vi "Planner_Creator.vi"(8 "error in (no error)":errorcluster) -> (0 "error out":errorcluster)   [LabVIEW 2017]
uses:
  <vilib>/Utility/file.llb/Read Delimited Spreadsheet (string).vi
  <vilib>/Utility/file.llb/Write Delimited Spreadsheet (string).vi
  <vilib>/Utility/config.llb/NI_LVConfig.lvlib
panel:
  out "SECTION 2":T1
  out "SECTION 1":T2
  in  "SECTION No":string(combo)
  in  "Delete Button":bool
  in  "Save Button":bool
  in  "Qty":u16=1 min=1 max=90 step=1
  in  "HOME":bool
  in  "UPDATE TABLE":bool
  in  "FG CAT No":string(combo)
  # "Plan Creater"
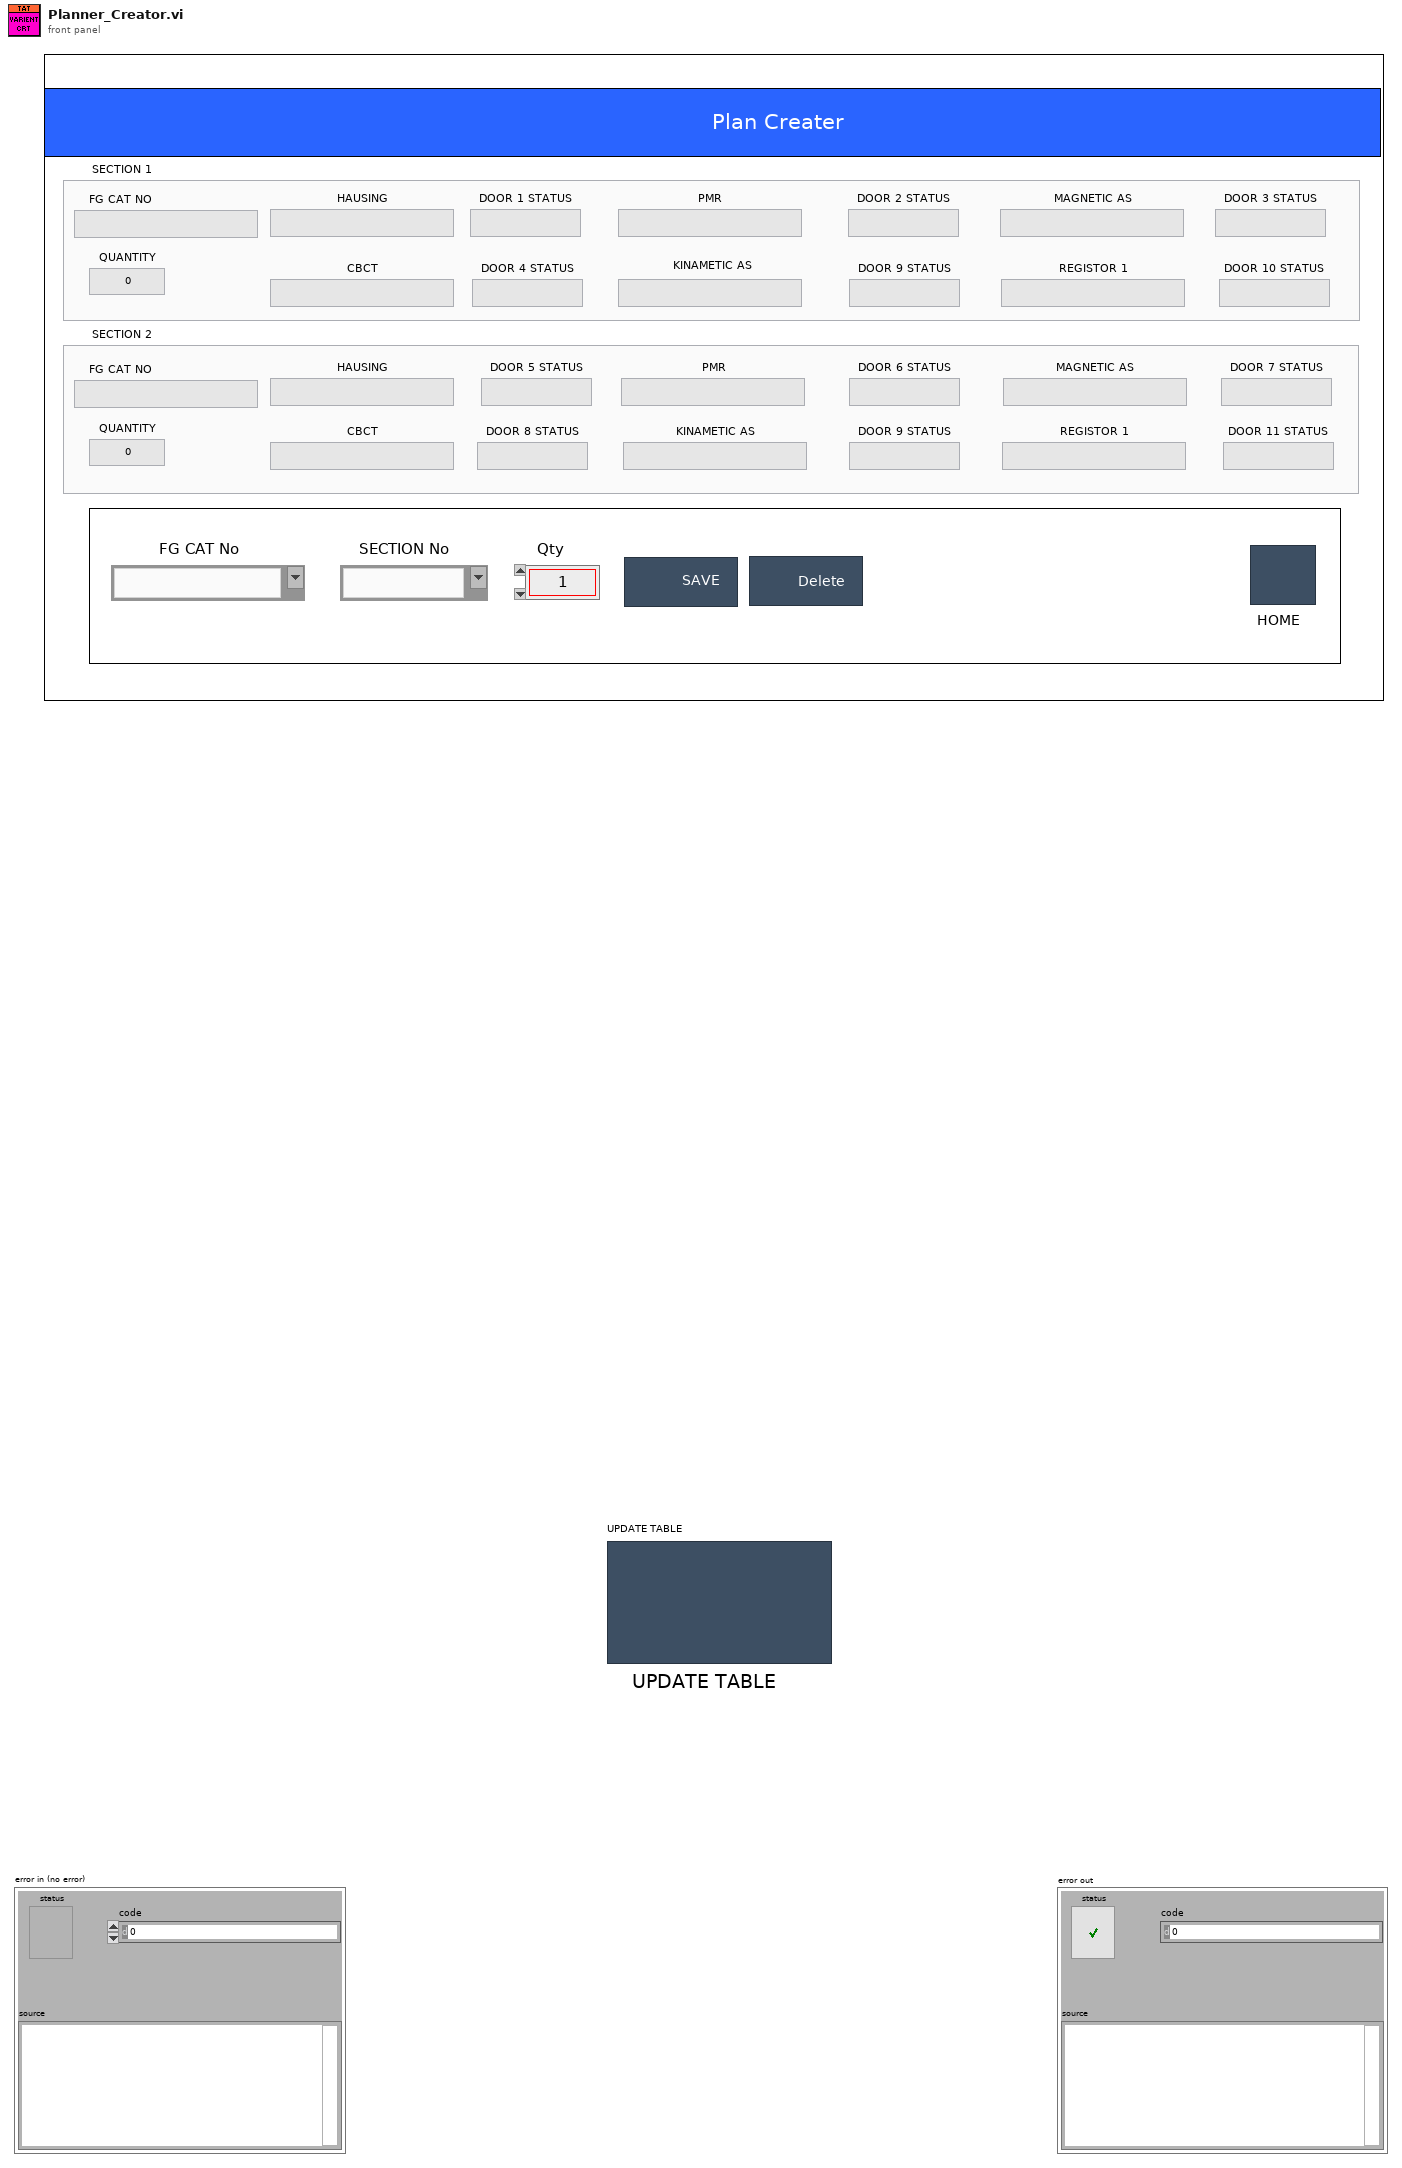
[diagram p1: front panel]
types:
  T1 = cluster{"FG CAT NO":string, "HAUSING":string, "DOOR 5 STATUS":string, "PMR":string, "DOOR 6 STATUS":string, "MAGNETIC AS":string, "DOOR 7 STATUS":string, "CBCT":string, "DOOR 8 STATUS":string, "KINAMETIC AS":string, "DOOR 9 STATUS":string, "REGISTOR 1":string, "DOOR 11 STATUS":string, "QUANTITY":u16}
  T2 = cluster{"FG CAT NO":string, "HAUSING":string, "DOOR 1 STATUS":string, "PMR":string, "DOOR 2 STATUS":string, "MAGNETIC AS":string, "DOOR 3 STATUS":string, "CBCT":string, "DOOR 4 STATUS":string, "KINAMETIC AS":string, "DOOR 9 STATUS":string, "REGISTOR 1":string, "DOOR 10 STATUS":string, "QUANTITY":u16}
  T3 = enum32{"invalid app kind", "Development System", "Run Time System", "Student Edition", "Embedded LabVIEW", "Evaluation", "Custom"}
  T4 = typedef "NI_LVConfig.lvlib/Config Data RefNum.ctl" = refnum<k1>
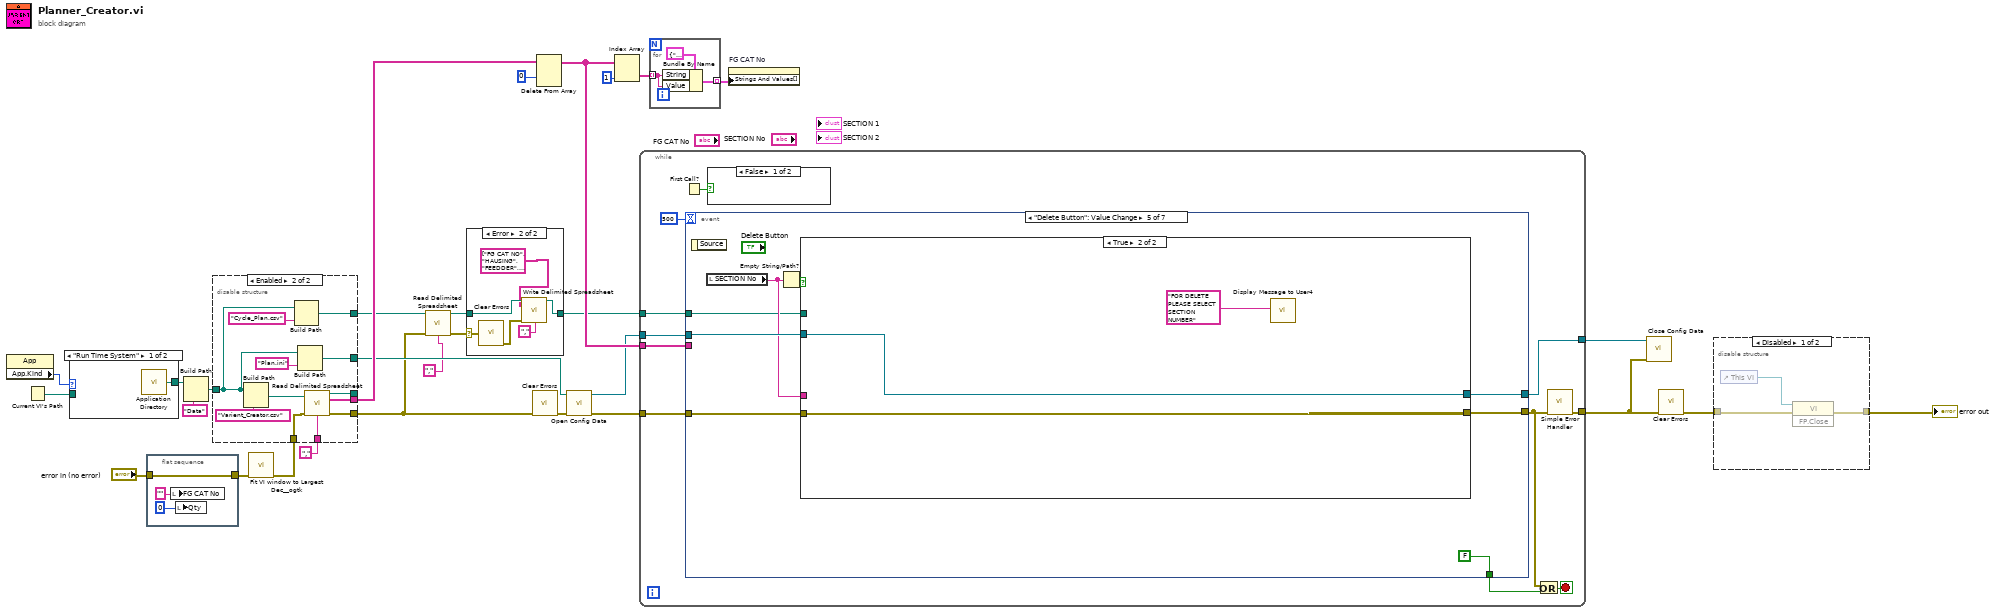
[diagram p0: block diagram]
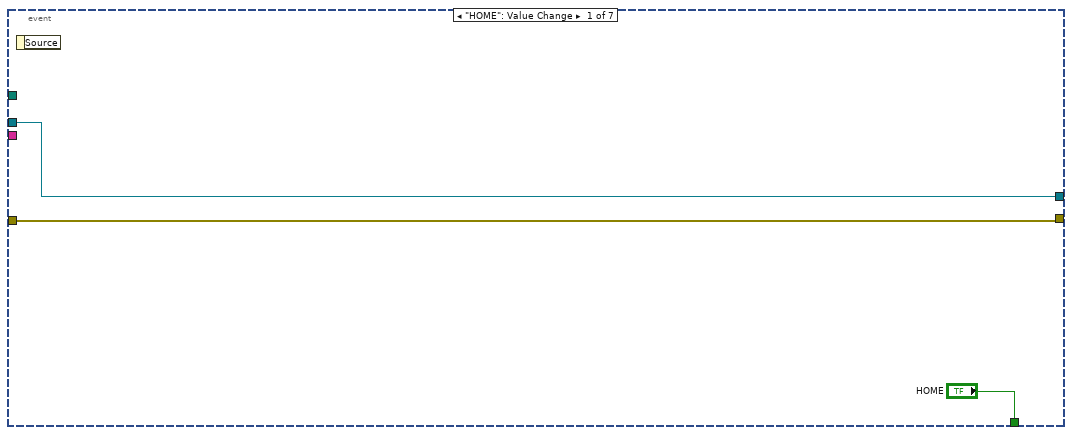
[diagram p4: hidden frame]
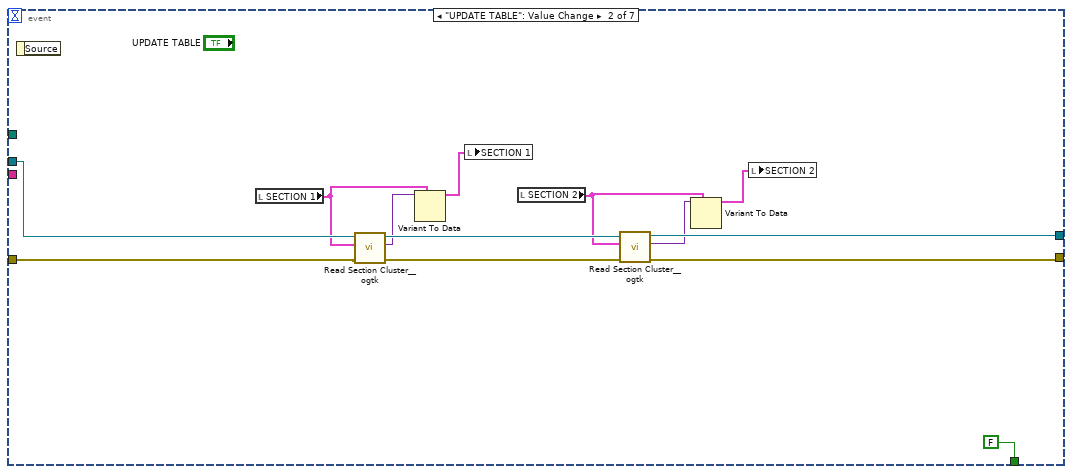
[diagram p5: hidden frame]
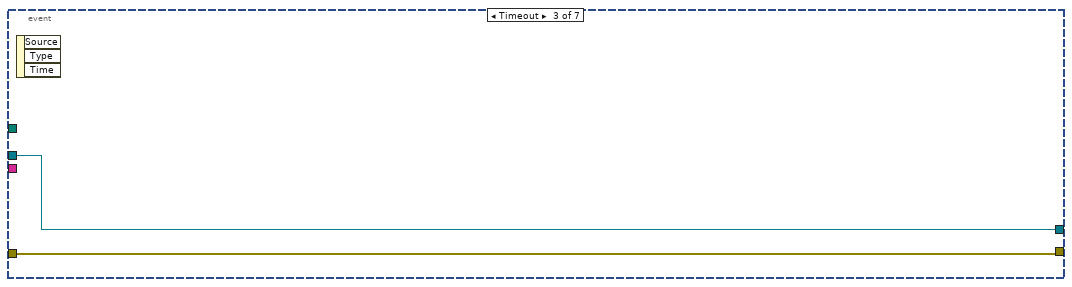
[diagram p6: hidden frame]
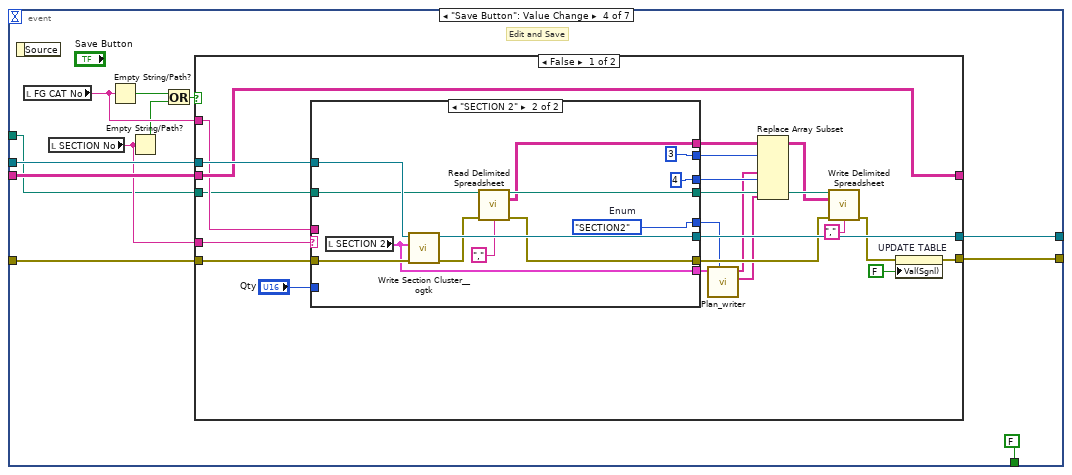
[diagram p7: hidden frame]
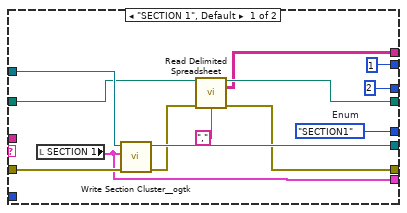
[diagram p8: hidden frame]
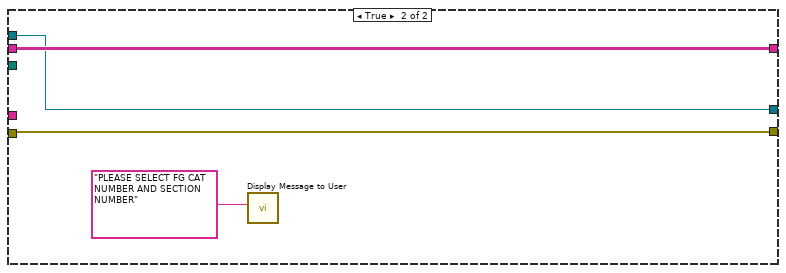
[diagram p9: hidden frame]
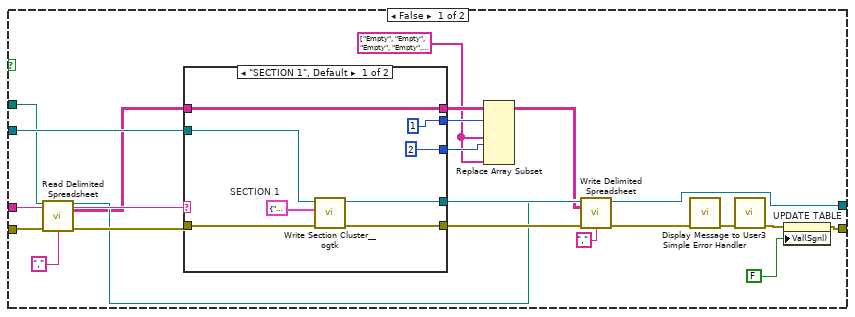
[diagram p10: hidden frame]
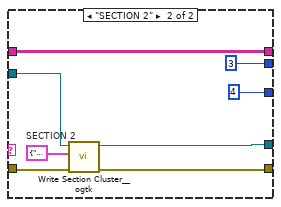
[diagram p11: hidden frame]
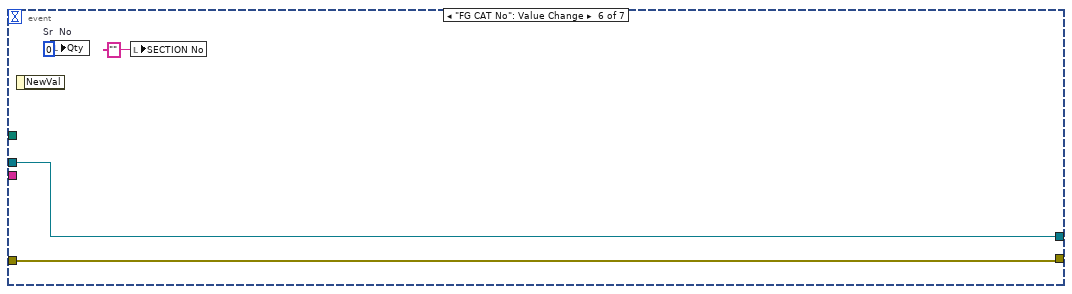
[diagram p12: hidden frame]
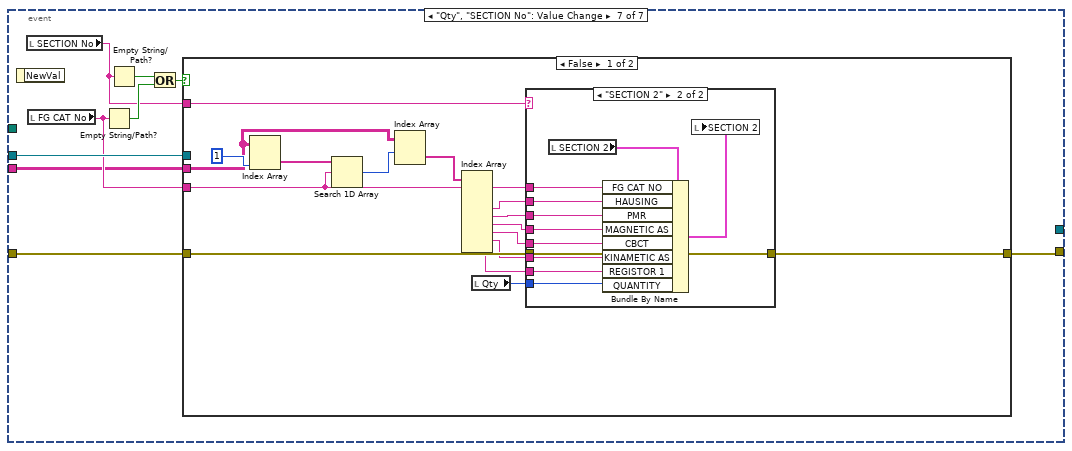
[diagram p13: hidden frame]
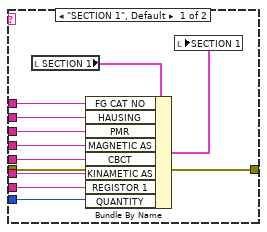
[diagram p14: hidden frame]
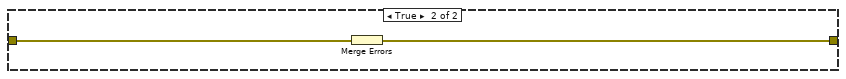
[diagram p15: hidden frame]
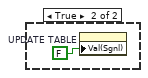
[diagram p16: hidden frame]
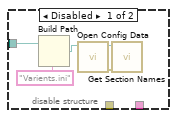
[diagram p17: hidden frame]
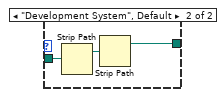
[diagram p18: hidden frame]
diagram:
  n1 = property class="App"() -> ("App.Kind"=w23:T3)  [unwired: 2 in, 2 out]
  n2 = Current VI's Path() -> (path=w24:path)
  n3 = case shown="\"Run Time System\"" w23 {
    tunnel: w24 -> [_ w32]
    tunnel: [w30 w31] -> w20
    frame "Run Time System" {
      n4 = call <vilib>:"Application Directory.vi"() -> ("Application Directory"=w30:path)
    }
    frame "Development System", Default {
      n5 = Strip Path(path=w32) -> (stripped path=w33:path)  [unwired: 1 out]
      n6 = Strip Path(path=w33) -> (stripped path=w31:path)  [unwired: 1 out]
    }
  }
  n7 = flat-sequence {
    tunnel: [w36] -> w25
    tunnel: "error in (no error)" -> [w36]
    frame #0 {
      n8 = local write "FG CAT No"("" ("PART NUMBER")) -> ()
      n9 = local write "Qty"(u16 0 ("BATCH SIZE")) -> ()
    }
  }
  n10 = Build Path(base path=w20, name or relative path="Data") -> (appended path=w21:path)
  n11 = call <userlib>:"Fit VI window to Largest Dec__ogtk.vi"("error in (no error)"=w25) -> ("error out"=w19:errorcluster)  [unwired: 5 in, 1 out]
  n12 = disable-structure shown="Enabled" {
    disable-tunnel: w21 -> [w37 w43]
    disable-tunnel: w19 -> [_ w51]
    disable-tunnel: [_ w50] -> w17
    disable-tunnel: [_ w49] -> _
    disable-tunnel: [_ w48] -> w6
    disable-tunnel: "," -> [_ w47]
    disable-tunnel: [_ w45] -> w11
    disable-tunnel: [_ w42] -> w5
    frame Disabled {
      n13 = Build Path(base path=w37, name or relative path="Varients.ini") -> (appended path=w41:path)
      n14 = call <vilib>:"Open Config Data.vi"("configuration file path"=w41) -> ("error out"=w38:errorcluster, "refnum"=w39:T4)  [unwired: 8 in, 1 out]
      n15 = call <vilib>:"Get Section Names.vi"("error in (no error)"=w38, "refnum"=w39) -> ()  [unwired: 7 in, 3 out]
    }
    frame Enabled {
      n16 = Build Path(base path=w43, name or relative path="Varient_Creator.csv") -> (appended path=w52:path)
      n17 = Build Path(base path=w43, name or relative path="Cycle_Plan.csv") -> (appended path=w42:path)
      n18 = Build Path(base path=w43, name or relative path="Plan.ini") -> (appended path=w45:path)
      n19 = call-poly <vilib>:"Read Delimited Spreadsheet.vi"("file path (dialog if empty)"=w52, "error in (no error)"=w51, "delimiter (\\t)"=w47) -> ("new file path (Not A Path if cancelled)"=w49:path, "all rows"=w50:string[][], "error out"=w48:errorcluster)  [unwired: 7 in, 3 out]
    }
  }
  n20 = call-poly <vilib>:"Read Delimited Spreadsheet.vi"("file path (dialog if empty)"=w5, "error in (no error)"=w6, "delimiter (\\t)"=",") -> ("new file path (Not A Path if cancelled)"=w1:path, "error out"=w3:errorcluster)  [unwired: 7 in, 4 out]
  n21 = case shown="Error" w3 {
    selector: w3 -> [_ w57]
    tunnel: [w54 w58] -> w2
    tunnel: w1 -> [w54 w59]
    frame No Error {
    }
    frame Error {
      n22 = call <vilib>:"Clear Errors.vi"("error in (no error)"=w57) -> ("error out"=w56:errorcluster)  [unwired: 5 in, 1 out]
      n23 = call-poly <vilib>:"Write Delimited Spreadsheet.vi"("file path (dialog if empty)"=w59, "2D data"=string[][] [["FG CAT NO", "HAUSING", "FEEDDER", "HAUSING_QR_CODE", "DOOR", "PMR", "FEEDDER", "PMR_QR_CODE", "DOOR", "MAGNETIC AS", "FEEDDER", "MAGNETIC AS_QR_CODE", "DOOR", "CBCT", "FEEDDER", "CBCT_QR_CODE", "DOOR", "KINAMETIC AS", "FEEDDER", "KINAMETIC AS_QR_CODE", "DOOR", "REGISTOR 1", "FEEDDER", "REGISTOR 1_QR_CODE", "DOOR", "QTY", "QTY_DONE"], ["Empty", "Empty", "Empty", "Empty", "Empty", "Empty", "Empty", "Empty", "Empty", "Empty", "Empty", "Empty", "Empty", "Empty", "Empty", "Empty", "Empty", "Empty", "Empty", "Empty", "Empty", "Empty", "Empty", "Empty", "Empty", "Empty", "Empty"], ["Empty", "Empty", "Empty", "Empty", "Empty", "Empty", "Empty", "Empty", "Empty", "Empty", "Empty", "Empty", "Empty", "Empty", "Empty", "Empty", "Empty", "Empty", "Empty", "Empty", "Empty", "Empty", "Empty", "Empty", "Empty", "Empty", "Empty"], ["Empty", "Empty", "Empty", "Empty", "Empty", "Empty", "Empty", "Empty", "Empty", "Empty", "Empty", "Empty", "Empty", "Empty", "Empty", "Empty", "Empty", "Empty", "Empty", "Empty", "Empty", "Empty", "Empty", "Empty", "Empty", "Empty", "Empty"], ["Empty", "Empty", "Empty", "Empty", "Empty", "Empty", "Empty", "Empty", "Empty", "Empty", "Empty", "Empty", "Empty", "Empty", "Empty", "Empty", "Empty", "Empty", "Empty", "Empty", "Empty", "Empty", "Empty", "Empty", "Empty", "Empty", "Empty"]], "error in (no error)"=w56, "delimiter (\\t)"=",") -> ("new file path (Not A Path if cancelled)"=w58:path)  [unwired: 10 in, 1 out]
    }
  }
  n24 = call <vilib>:"Clear Errors.vi"("error in (no error)"=w6) -> ("error out"=w9:errorcluster)  [unwired: 5 in, 1 out]
  n25 = Delete From Array(array=w17, index (row)=0) -> (array with subset deleted=w12:string[][])  [unwired: 2 in, 1 out]
  n26 = call <vilib>:"Open Config Data.vi"("error in (no error)"=w9, "configuration file path"=w11) -> ("error out"=w8:errorcluster, "refnum"=w10:T4)  [unwired: 7 in, 1 out]
  n27 = Index Array(array=w12, index (col)=1) -> (element=w14:string[])  [unwired: 1 in]
  n28 = while {
    tunnel: [w66] -> w27
    tunnel: w8 -> [w68]
    tunnel: w12 -> [w64]
    tunnel: w10 -> [w63]
    tunnel: [w62] -> w7
    tunnel: w2 -> [w61]
    stop <- w70 stop-if-true
    n29 = First Call?() -> (First Call?: T/F=w69:bool)
    n30 = event shown="[4] \"Delete Button\": Value Change" {
      selector: _ -> [_ _ _ _ _ _ _]
      dyn-events: _ -> [_ _ _ _ _ _ _]
      timeout: 500 -> [_ _ _ _ _ _ _]
      tunnel: ["HOME" FALSE ("stop") _ FALSE ("stop") FALSE ("stop") _ _] -> w71
      tunnel: [w73 w84 w89 w99 w159 w204 w213] -> w67
      tunnel: w68 -> [w73 w85 w89 w98 w158 w204 w214]
      tunnel: w64 -> [_ _ _ w97 _ _ w206]
      tunnel: w63 -> [w72 w82 w88 w93 w157 w202 w209]
      tunnel: [w72 w81 w88 w91 w156 w202 _] -> w62
      tunnel: w61 -> [_ _ _ w90 w154 _ _]
      event "HOME": Value Change {
        n31 = event-data() -> ()  [unwired: 1 in, 1 out]
      }
      event "UPDATE TABLE": Value Change {
        n32 = event-data() -> ()  [unwired: 1 in, 1 out]
        n33 = local read "SECTION 1"() -> (w80:T2)
        n34 = call <userlib>:"Read Section Cluster__ogtk.vi"("error in (no error)"=w85, "Section Formatted Cluster Type"=w80, "refnum"=w82) -> ("error out"=w86:errorcluster, "Section Formatted Cluster"=w79:variant, "dup refnum"=w83:T4)  [unwired: 4 in, 2 out]
        n35 = Variant To Data(type=w80, Variant=w79) -> (data=w75:T2)  [unwired: 1 in, 1 out]
        n36 = local write "SECTION 1"(w75) -> ()
        n37 = local read "SECTION 2"() -> (w78:T1)
        n38 = call <userlib>:"Read Section Cluster__ogtk.vi"("error in (no error)"=w86, "Section Formatted Cluster Type"=w78, "refnum"=w83) -> ("error out"=w84:errorcluster, "Section Formatted Cluster"=w77:variant, "dup refnum"=w81:T4)  [unwired: 4 in, 2 out]
        n39 = Variant To Data(type=w78, Variant=w77) -> (data=w76:T1)  [unwired: 1 in, 1 out]
        n40 = local write "SECTION 2"(w76) -> ()
      }
      event Timeout {
        n41 = event-data() -> ()  [unwired: 1 in, 3 out]
      }
      event "Save Button": Value Change {
        # "Edit and Save"
        n42 = event-data() -> ()  [unwired: 1 in, 1 out]
        n43 = local read "FG CAT No"() -> (w100:string)
        n44 = local read "SECTION No"() -> (w92:string)
        n45 = Empty String/Path?(string/path=w100) -> (empty?=w95:bool)
        n46 = Empty String/Path?(string/path=w92) -> (empty?=w96:bool)
        n47 = Or(x=w95, y=w96) -> (x .or. y?=w94:bool)
        n48 = case shown="False" w94 {
          tunnel: [w122 w152] -> w99
          tunnel: w100 -> [w118 _]
          tunnel: w98 -> [w120 w152]
          tunnel: w97 -> [w119 w151]
          tunnel: w93 -> [w121 w150]
          tunnel: [w119 w151] -> _
          tunnel: w92 -> [w117 _]
          tunnel: [w115 w150] -> w91
          tunnel: w90 -> [w114 _]
          frame False {
            n49 = case shown="\"SECTION 2\"" w117 {
              tunnel: w121 -> [w135 w148]
              tunnel: w120 -> [w136 w147]
              tunnel: [w130 w145] -> w112
              tunnel: w118 -> [_ _]
              tunnel: "Qty" -> [_ _]
              tunnel: [w134 w149] -> w115
              tunnel: w114 -> [w132 w144]
              tunnel: [w129 w143] -> w113
              tunnel: [w128 w141] -> w109
              tunnel: [1 ("disabled index (col)") 3 ("disabled index (col)")] -> w107
              tunnel: [2 ("disabled index (col)") 4 ("disabled index (col)")] -> w106
              tunnel: [w125 w138] -> w105
              tunnel: [w124 w137] -> w102
              frame "SECTION 1", Default {
                w124 = enum16{"SECTION1", "SECTION2"}."SECTION1"  # Enum
                n50 = local read "SECTION 1"() -> (w125:T2)
                n51 = call <userlib>:"Write Section Cluster__ogtk.vi"("error in (no error)"=w136, "Section Formatted Cluster"=w125, "refnum"=w135) -> ("error out"=w131:errorcluster, "dup refnum"=w134:T4)  [unwired: 7 in]
                n52 = call-poly <vilib>:"Read Delimited Spreadsheet.vi"("file path (dialog if empty)"=w132, "error in (no error)"=w131, "delimiter (\\t)"=",") -> ("new file path (Not A Path if cancelled)"=w129:path, "all rows"=w128:string[][], "error out"=w130:errorcluster)  [unwired: 7 in, 3 out]
              }
              frame "SECTION 2" {
                w137 = enum16{"SECTION1", "SECTION2"}."SECTION2"  # Enum
                n53 = local read "SECTION 2"() -> (w138:T1)
                n54 = call <userlib>:"Write Section Cluster__ogtk.vi"("error in (no error)"=w147, "Section Formatted Cluster"=w138, "refnum"=w148) -> ("error out"=w146:errorcluster, "dup refnum"=w149:T4)  [unwired: 7 in]
                n55 = call-poly <vilib>:"Read Delimited Spreadsheet.vi"("file path (dialog if empty)"=w144, "error in (no error)"=w146, "delimiter (\\t)"=",") -> ("new file path (Not A Path if cancelled)"=w143:path, "all rows"=w141:string[][], "error out"=w145:errorcluster)  [unwired: 7 in, 3 out]
              }
            }
            n56 = call "Plan_writer.vi"("Enum"=w102, "SECTION IN"=w105) -> ("Section Second 45"=w103:string[], "Section first 45"=w104:string[])  [unwired: 8 in]
            n57 = Replace Array Subset(array=w109, new element #1=w104, index (row) #1=w107, new element #2=w103, index (row) #2=w106) -> (w108:string[][])  [unwired: 2 in]
            n58 = call-poly <vilib>:"Write Delimited Spreadsheet.vi"("file path (dialog if empty)"=w113, "2D data"=w108, "error in (no error)"=w112, "delimiter (\\t)"=",") -> ("error out"=w111:errorcluster)  [unwired: 10 in, 1 out]
            n59 = property on="UPDATE TABLE" class="Bool (strict)"(error in=w111, "Val(Sgnl)"=FALSE) -> (error out=w122:errorcluster)  [unwired: 1 in, 1 out]
          }
          frame True {
            n60 = call "Display Message to User"("Message"="PLEASE SELECT FG CAT NUMBER AND SECTION NUMBER") -> ()  [unwired: 9 in, 2 out]
          }
        }
      }
      event "Delete Button": Value Change {
        n61 = event-data() -> ()  [unwired: 1 in, 1 out]
        n62 = local read "SECTION No"() -> (w155:string)
        n63 = Empty String/Path?(string/path=w155) -> (empty?=w160:bool)
        n64 = case shown="True" w160 {
          tunnel: [w181 w200] -> w159
          tunnel: w158 -> [w175 w200]
          tunnel: w157 -> [w178 w199]
          tunnel: [w177 w199] -> w156
          tunnel: w155 -> [w176 _]
          tunnel: w154 -> [w172 _]
          frame False {
            w163 = string[] ["Empty", "Empty", "Empty", "Empty", "Empty", "Empty", "Empty", "Empty", "Empty", "Empty", "Empty", "Empty", "Empty", "Empty", "Empty", "Empty", "Empty", "Empty", "Empty", "Empty", "Empty", "Empty", "Empty", "Empty", "Empty", "Empty", "Empty"]
            n65 = call-poly <vilib>:"Read Delimited Spreadsheet.vi"("file path (dialog if empty)"=w172, "error in (no error)"=w175, "delimiter (\\t)"=",") -> ("new file path (Not A Path if cancelled)"=w168:path, "all rows"=w166:string[][], "error out"=w174:errorcluster)  [unwired: 7 in, 3 out]
            n66 = case shown="\"SECTION 1\", Default" w176 {
              tunnel: w174 -> [w190 w196]
              tunnel: [w189 w198] -> w170
              tunnel: [w188 w197] -> w177
              tunnel: w178 -> [w187 w195]
              tunnel: [w185 w193] -> w167
              tunnel: w166 -> [w185 w193]
              tunnel: [1 ("disabled index (col)") 3 ("disabled index (col)")] -> w165
              tunnel: [2 ("disabled index (col)") 4 ("disabled index (col)")] -> w164
              frame "SECTION 1", Default {
                w186 = T2 {"FG CAT NO"="", "HAUSING"="", "DOOR 1 STATUS"="PENDING", "PMR"="", "DOOR 2 STATUS"="PENDING", "MAGNETIC AS"="", "DOOR 3 STATUS"="PENDING", "CBCT"="", "DOOR 4 STATUS"="PENDING", "KINAMETIC AS"="", "DOOR 9 STATUS"="PENDING", "REGISTOR 1"="", "DOOR 10 STATUS"="PENDING", "QUANTITY"=0}  # SECTION 1
                n67 = call <userlib>:"Write Section Cluster__ogtk.vi"("error in (no error)"=w190, "Section Formatted Cluster"=w186, "refnum"=w187) -> ("error out"=w189:errorcluster, "dup refnum"=w188:T4)  [unwired: 7 in]
              }
              frame "SECTION 2" {
                w194 = T1 {"FG CAT NO"="", "HAUSING"="", "DOOR 5 STATUS"="PENDING", "PMR"="", "DOOR 6 STATUS"="PENDING", "MAGNETIC AS"="", "DOOR 7 STATUS"="PENDING", "CBCT"="", "DOOR 8 STATUS"="PENDING", "KINAMETIC AS"="", "DOOR 9 STATUS"="PENDING", "REGISTOR 1"="", "DOOR 11 STATUS"="PENDING", "QUANTITY"=0}  # SECTION 2
                n68 = call <userlib>:"Write Section Cluster__ogtk.vi"("error in (no error)"=w196, "Section Formatted Cluster"=w194, "refnum"=w195) -> ("error out"=w198:errorcluster, "dup refnum"=w197:T4)  [unwired: 7 in]
              }
            }
            n69 = Replace Array Subset(array=w167, new element #1=w163, index (row) #1=w165, new element #2=w163, index (row) #2=w164) -> (w162:string[][])  [unwired: 2 in]
            n70 = call-poly <vilib>:"Write Delimited Spreadsheet.vi"("file path (dialog if empty)"=w168, "2D data"=w162, "error in (no error)"=w170, "delimiter (\\t)"=",") -> ("error out"=w169:errorcluster)  [unwired: 10 in, 1 out]
            n71 = call <vilib>:"Simple Error Handler.vi"("error in (no error)"=w169) -> ("error out"=w180:errorcluster)  [unwired: 4 in, 4 out]
            n72 = call "Display Message to User3"("error in (no error)"=w180) -> ("error out"=w179:errorcluster)  [unwired: 9 in, 1 out]
            n73 = property on="UPDATE TABLE" class="Bool (strict)"(error in=w179, "Val(Sgnl)"=FALSE) -> (error out=w181:errorcluster)  [unwired: 1 in, 1 out]
          }
          frame True {
            n74 = call "Display Message to User4"("Message"="FOR DELETE PLEASE SELECT SECTION NUMBER") -> ()  [unwired: 9 in, 2 out]
          }
        }
      }
      event "FG CAT No": Value Change {
        w205 = u16 0  # Sr  No
        n75 = event-data() -> ()  [unwired: 1 in, 1 out]
        n76 = local write "Qty"(w205) -> ()
        n77 = local write "SECTION No"("") -> ()
      }
      event "Qty", "SECTION No": Value Change {
        n78 = event-data() -> ()  [unwired: 1 in, 1 out]
        n79 = local read "SECTION No"() -> (w207:string)
        n80 = local read "FG CAT No"() -> (w208:string)
        n81 = Empty String/Path?(string/path=w208) -> (empty?=w211:bool)
        n82 = Empty String/Path?(string/path=w207) -> (empty?=w212:bool)
        n83 = Or(x=w212, y=w211) -> (x .or. y?=w210:bool)
        n84 = case shown="False" w210 {
          tunnel: w214 -> [w230 w254]
          tunnel: [w229 w253] -> w213
          tunnel: w209 -> [_ _]
          tunnel: w207 -> [w228 _]
          tunnel: w208 -> [w225 _]
          tunnel: w206 -> [w222 _]
          frame False {
            n85 = Index Array(array=w222, index (col)=1) -> (element=w224:string[])  [unwired: 1 in]
            n86 = Search 1D Array(1D array=w224, element=w225) -> (index of element=w223:i32)  [unwired: 1 in]
            n87 = Index Array(array=w222, index (row)=w223) -> (element=w221:string[])  [unwired: 1 in]
            n88 = Index Array(array=w221) -> (element #3=w220:string, element #4=w219:string, element #5=w218:string, element #6=w217:string, element #7=w216:string, element #8=w215:string)  [unwired: 8 in, 2 out]
            n89 = local read "Qty"() -> (w227:u16)
            n90 = case shown="\"SECTION 2\"" w228 {
              tunnel: w230 -> [w241 w252]
              tunnel: [w241 w252] -> w229
              tunnel: w225 -> [w239 w248]
              tunnel: w227 -> [w238 w249]
              tunnel: w220 -> [w231 w247]
              tunnel: w219 -> [w232 w246]
              tunnel: w218 -> [w233 w245]
              tunnel: w217 -> [w234 w244]
              tunnel: w216 -> [w235 w243]
              tunnel: w215 -> [w236 w242]
              frame "SECTION 1", Default {
                n91 = local read "SECTION 1"() -> (w240:T2)
                n92 = Bundle By Name(cluster=w240, "FG CAT NO"=w239, "HAUSING"=w231, "PMR"=w232, "MAGNETIC AS"=w233, "CBCT"=w234, "KINAMETIC AS"=w235, "REGISTOR 1"=w236, "QUANTITY"=w238) -> (w237:T2)
                n93 = local write "SECTION 1"(w237) -> ()
              }
              frame "SECTION 2" {
                n94 = local read "SECTION 2"() -> (w251:T1)
                n95 = Bundle By Name(cluster=w251, "FG CAT NO"=w248, "HAUSING"=w247, "PMR"=w246, "MAGNETIC AS"=w245, "CBCT"=w244, "KINAMETIC AS"=w243, "REGISTOR 1"=w242, "QUANTITY"=w249) -> (w250:T1)
                n96 = local write "SECTION 2"(w250) -> ()
              }
            }
          }
          frame True {
            n97 = Merge Errors(w254) -> (w253:errorcluster)
          }
        }
      }
    }
    n98 = case shown="False" w69 {
      frame False {
      }
      frame True {
        n99 = property on="UPDATE TABLE" class="Bool (strict)"("Val(Sgnl)"=FALSE) -> ()  [unwired: 2 in, 2 out]
      }
    }
    n100 = Or(x=w67, y=w71) -> (x .or. y?=w70:bool)
    n101 = call <vilib>:"Simple Error Handler.vi"("error in (no error)"=w67) -> ("error out"=w66:errorcluster)  [unwired: 4 in, 4 out]
  }
  n102 = for {
    tunnel: w14 -> [w257] mode=indexing
    tunnel: [w256] -> w13 mode=indexing
    n103 = Bundle By Name(cluster=cluster{"String":string, "Value":string} {"String"="", "Value"=""}, "String"=w257, "Value"=w257) -> (w256:cluster{"String":string, "Value":string})
  }
  n104 = property on="FG CAT No" class="CmbBox"("Strings And Values[]"=w13) -> ()  [unwired: 2 in, 2 out]
  n105 = call <vilib>:"Close Config Data.vi"("error in (no error)"=w27, "refnum"=w7) -> ()  [unwired: 8 in, 2 out]
  n106 = call <vilib>:"Clear Errors.vi"("error in (no error)"=w27) -> ("error out"=w29:errorcluster)  [unwired: 5 in, 1 out]
  n107 = disable-structure shown="Disabled" {
    disable-tunnel: w29 -> [w261 w262]
    disable-tunnel: [w260 w262] -> w28
    frame Disabled {
      n108 = control-ref of="This VI"() -> (w259:refnum<vi>)
      n109 = invoke class="VI" method="FP.Close"(reference=w259, error in=w261) -> (error out=w260:errorcluster)  [unwired: 1 in, 2 out]
    }
    frame Enabled {
    }
  }
  "error out" <- w28
